vi "toXML.vi"(8 "error in (no error)":errorcluster, 11 "Sequence in":refnum<class "Sequence.lvclass">) -> (0 "error out":errorcluster, 2 "xmlNode":refnum<class "xmlNode.lvclass">, 3 "Sequence out":refnum<class "Sequence.lvclass">)   [LabVIEW 2009, in "Tools.lvlib" / "Sequencing.lvlib" / "Sequence.lvclass"]
uses:
  Sequence.lvclass
  xmlNode/xmlNode.lvclass
  Sequence.lvclass/Sequence.ctl
  Points/Point/Point.lvclass
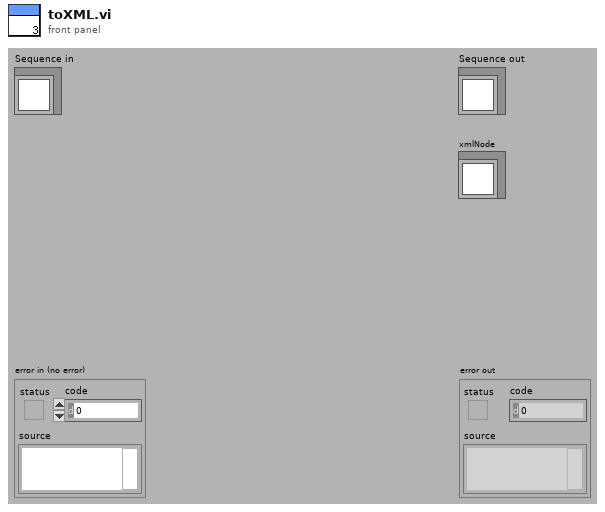
[diagram p1: front panel]
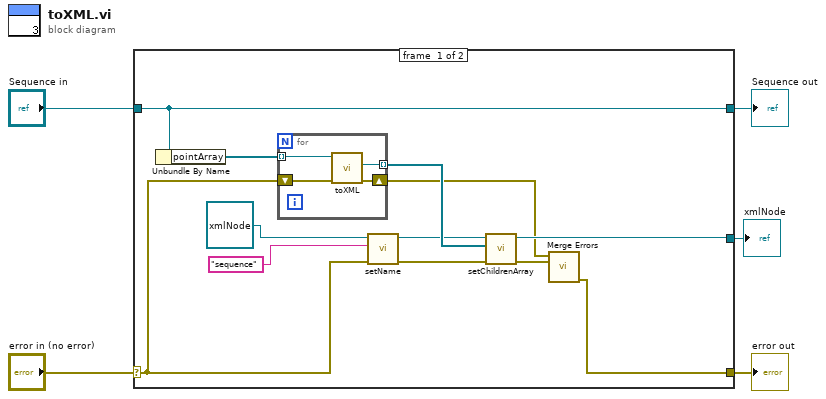
[diagram p0: block diagram]
diagram:
  n1 = case shown="No Error" "error in (no error)" {
    selector: "error in (no error)" -> [w10 w23]
    tunnel: [w6 w23] -> w4
    tunnel: [w17 w22] -> w2
    tunnel: "Sequence in" -> [w17 w22]
    tunnel: [w9 _] -> w1
    frame #0 {
      n2 = Unbundle By Name(w17) -> ("pointArray"=w16:refnum<class "Point.lvclass">[])
      n3 = for {
        tunnel: w16 -> [w21] mode=indexing
        shift-right: [w19] -> w8
        shift-left: w10 -> [w20]
        tunnel: [w18] -> w15 mode=indexing
        n4 = call-dynamic "toXML.vi"("error in (no error)"=w20, "Point in"=w21) -> ("error out"=w19:errorcluster, "xmlNode"=w18:refnum<class "xmlNode.lvclass">)  [unwired: 7 in, 1 out]
      }
      n5 = call-dynamic "setName.vi"("error in (no error)"=w10, "name"="sequence", "xmlNode.lvclass in"=refnum<class "xmlNode.lvclass"> refnum ("Tools.lvlib:xml.lvlib:xmlNode.lvclass")) -> ("error out"=w13:errorcluster, "xmlNode.lvclass out"=w14:refnum<class "xmlNode.lvclass">)  [unwired: 7 in]
      n6 = call-dynamic "setChildrenArray.vi"("error in (no error)"=w13, "Children"=w15, "xmlNode.lvclass in"=w14) -> ("error out"=w7:errorcluster, "xmlNode.lvclass out"=w9:refnum<class "xmlNode.lvclass">)  [unwired: 7 in]
      n7 = call <vilib>:"Merge Errors.vi"("error in 2 (no error)"=w7, "error in 1 (no error)"=w8) -> ("error out"=w6:errorcluster)  [unwired: 5 in]
    }
    frame #1 {
    }
  }
  "error out" <- w4
  "Sequence out" <- w2
  "xmlNode" <- w1
